vi "Lab Panel V5.24.vi"() -> ()   [LabVIEW 2013] (continued)
            n2217 = Equal?(x=w3930, y=1) -> (x = y?=w3916:bool)
            n2218 = Equal?(x=w3930, y=w3931) -> (x = y?=w3915:bool)
            n2219 = stacked-sequence {
              tunnel: w3929 -> [w3939 _ _ _ _ _ _ _ _ _]
              tunnel: w3928 -> [_ w4015 _ _ _ _ _ _ _ _]
              tunnel: w3927 -> [_ _ w4095 _ _ _ _ _ _ _]
              tunnel: w3926 -> [_ _ _ w4175 _ _ _ _ _ _]
              tunnel: w3925 -> [_ _ _ _ w4255 _ _ _ _ _]
              tunnel: w3924 -> [_ _ _ _ _ w4335 _ _ _ _]
              tunnel: w3923 -> [_ _ _ _ _ _ w4415 _ _ _]
              tunnel: w3922 -> [_ _ _ _ _ _ _ w4495 _ _]
              tunnel: w3921 -> [_ _ _ _ _ _ _ _ w4575 _]
              tunnel: w3920 -> [_ _ _ _ _ _ _ _ _ w4655]
              tunnel: w3917 -> [w3938 w4019 w4099 w4179 w4259 w4339 w4419 w4499 w4579 w4659]
              tunnel: w3916 -> [w3937 w4018 w4098 w4178 w4258 w4338 w4418 w4498 w4578 w4658]
              tunnel: w3915 -> [w3936 w4017 w4097 w4177 w4257 w4337 w4417 w4497 w4577 w4657]
              tunnel: w3914 -> [w3935 w4016 w4096 w4176 w4256 w4336 w4416 w4496 w4576 w4656]
              frame #0 {
                n2220 = case shown="True" w3939 {
                  tunnel: w3938 -> [_ w3944]
                  tunnel: w3937 -> [_ w3943]
                  tunnel: w3936 -> [_ w3941]
                  tunnel: w3935 -> [_ w3940]
                  frame False {
                  }
                  frame True {
                    n2221 = local read "DISP LAB01-1"() -> (w3945:T4)
                    n2222 = local read "SIG LAB01-1"() -> (w3946:T2)
                    n2223 = local read "ON L01-1"() -> (w3942:cluster{"amps":dbl, "volts":dbl, "pf":dbl})
                    n2224 = Unbundle(w3946) -> ("AMPS"=w3952:dbl, "VOLTS"=w3950:dbl, "PF"=w3949:dbl, "Tmp Live"=w3948:dbl, "Tmp Neut"=w3951:dbl)
                    n2225 = Unbundle(w3945) -> ("CYCLE"=w3947:dbl)  [unwired: 2 out]
                    n2226 = stacked-sequence {
                      tunnel: w3952 -> [w3956 w3975]
                      tunnel: w3951 -> [_ w3974]
                      tunnel: w3950 -> [w3955 w3973]
                      tunnel: w3949 -> [w3954 w3972]
                      tunnel: w3948 -> [_ w3971]
                      tunnel: w3947 -> [_ w3970]
                      tunnel: w3944 -> [_ w3969]
                      tunnel: w3943 -> [w3957 _]
                      tunnel: w3942 -> [w3953 w3967]
                      tunnel: w3941 -> [_ w3968]
                      tunnel: w3940 -> [_ w3963]
                      frame #0 {
                        n2227 = case shown="True" w3957 {
                          tunnel: w3956 -> [_ w3962]
                          tunnel: w3955 -> [_ w3961]
                          tunnel: w3954 -> [_ w3960]
                          tunnel: w3953 -> [_ w3958]
                          frame False {
                          }
                          frame True {
                            n2228 = Bundle(cluster=w3958, "amps"=w3962, "volts"=w3961, "pf"=w3960) -> (w3959:cluster{"amps":dbl, "volts":dbl, "pf":dbl})
                            n2229 = local write "ON L01-1"(w3959) -> ()
                          }
                        }
                      }
                      frame #1 {
                        n2230 = Unbundle(w3967) -> ("amps"=w3966:dbl, "volts"=w3965:dbl, "pf"=w3964:dbl)
                        n2231 = case shown="True" w3968 {
                          tunnel: w3975 -> [_ w3976]
                          tunnel: w3974 -> [_ w4014]
                          tunnel: w3973 -> [_ _]
                          tunnel: w3972 -> [_ _]
                          tunnel: w3971 -> [_ w4013]
                          tunnel: w3970 -> [_ w4012]
                          tunnel: w3969 -> [_ w3980]
                          tunnel: w3966 -> [_ w3977]
                          tunnel: w3965 -> [_ w4009]
                          tunnel: w3964 -> [_ w4008]
                          tunnel: w3963 -> [_ w3978]
                          frame False {
                          }
                          frame True {
                            n2232 = local read "TDMS LAB01-1"() -> (w4011:refnum<k34>)
                            n2233 = Build Array(w4009) -> (w4005:dbl[])
                            n2234 = Build Array(w4008) -> (w4004:dbl[])
                            n2235 = Build Array(w4013) -> (w4003:dbl[])
                            n2236 = Build Array(w4014) -> (w4002:dbl[])
                            n2237 = Build Array(w3977) -> (w4007:dbl[])
                            n2238 = Build Array(w3976) -> (w4006:dbl[])
                            n2239 = Build Array(w4012) -> (w4001:dbl[])
                            n2240 = Build Array("AMPS ON", "AMPS OFF", "VOLTS", "PF", "TEMP Live", "TEMP Neut", "CYCLE") -> (w3985:string[])
                            n2241 = Bundle By Name("Y"=w4007, "t0"=w3978) -> (w4000:waveform(dbl))  [unwired: 1 in]
                            n2242 = Bundle By Name("Y"=w4006, "t0"=w3978) -> (w3999:waveform(dbl))  [unwired: 1 in]
                            n2243 = Bundle By Name("Y"=w4005, "t0"=w3978) -> (w3998:waveform(dbl))  [unwired: 1 in]
                            n2244 = Bundle By Name("Y"=w4004, "t0"=w3978) -> (w3997:waveform(dbl))  [unwired: 1 in]
                            n2245 = Bundle By Name("Y"=w4003, "t0"=w3978) -> (w3996:waveform(dbl))  [unwired: 1 in]
                            n2246 = Bundle By Name("Y"=w4002, "t0"=w3978) -> (w3995:waveform(dbl))  [unwired: 1 in]
                            n2247 = Bundle By Name("Y"=w4001, "t0"=w3978) -> (w3994:waveform(dbl))  [unwired: 1 in]
                            n2248 = Build Array(w4000, w3999, w3998, w3997, w3996, w3995, w3994) -> (w3993:waveform(dbl)[])
                            n2249 = TDMS Write(0:w4011, 5:"TEST VALUES", 7:w3985, 9:w3993) -> (4:w3984:refnum<k34>, 6:w3983:string, 15:w3982:errorcluster)  [unwired: 2 in, 1 out]
                            n2250 = TDMS Write(0:w3984, 5:w3983, 7:"TIME", 9:w3980, 11:w3982) -> (15:w3979:errorcluster)  [unwired: 1 in, 3 out]
                            n2251 = local write "data file error"(w3979) -> ()
                          }
                        }
                      }
                    }
                  }
                }
              }
              frame #1 {
                n2252 = case shown="True" w4015 {
                  tunnel: w4019 -> [_ w4024]
                  tunnel: w4018 -> [_ w4023]
                  tunnel: w4017 -> [_ w4021]
                  tunnel: w4016 -> [_ w4020]
                  frame False {
                  }
                  frame True {
                    n2253 = local read "DISP LAB01-2"() -> (w4025:T4)
                    n2254 = local read "SIG LAB01-2"() -> (w4026:T2)
                    n2255 = local read "ON L01-2"() -> (w4022:cluster{"amps":dbl, "volts":dbl, "pf":dbl})
                    n2256 = Unbundle(w4026) -> ("AMPS"=w4032:dbl, "VOLTS"=w4030:dbl, "PF"=w4029:dbl, "Tmp Live"=w4028:dbl, "Tmp Neut"=w4031:dbl)
                    n2257 = Unbundle(w4025) -> ("CYCLE"=w4027:dbl)  [unwired: 2 out]
                    n2258 = stacked-sequence {
                      tunnel: w4032 -> [w4036 w4055]
                      tunnel: w4031 -> [_ w4054]
                      tunnel: w4030 -> [w4035 w4053]
                      tunnel: w4029 -> [w4034 w4052]
                      tunnel: w4028 -> [_ w4051]
                      tunnel: w4027 -> [_ w4050]
                      tunnel: w4024 -> [_ w4049]
                      tunnel: w4023 -> [w4037 _]
                      tunnel: w4022 -> [w4033 w4047]
                      tunnel: w4021 -> [_ w4048]
                      tunnel: w4020 -> [_ w4043]
                      frame #0 {
                        n2259 = case shown="True" w4037 {
                          tunnel: w4036 -> [_ w4042]
                          tunnel: w4035 -> [_ w4041]
                          tunnel: w4034 -> [_ w4040]
                          tunnel: w4033 -> [_ w4038]
                          frame False {
                          }
                          frame True {
                            n2260 = Bundle(cluster=w4038, "amps"=w4042, "volts"=w4041, "pf"=w4040) -> (w4039:cluster{"amps":dbl, "volts":dbl, "pf":dbl})
                            n2261 = local write "ON L01-2"(w4039) -> ()
                          }
                        }
                      }
                      frame #1 {
                        n2262 = Unbundle(w4047) -> ("amps"=w4046:dbl, "volts"=w4045:dbl, "pf"=w4044:dbl)
                        n2263 = case shown="True" w4048 {
                          tunnel: w4055 -> [_ w4087]
                          tunnel: w4054 -> [_ w4094]
                          tunnel: w4053 -> [_ _]
                          tunnel: w4052 -> [_ _]
                          tunnel: w4051 -> [_ w4093]
                          tunnel: w4050 -> [_ w4092]
                          tunnel: w4049 -> [_ w4057]
                          tunnel: w4046 -> [_ w4089]
                          tunnel: w4045 -> [_ w4088]
                          tunnel: w4044 -> [_ w4086]
                          tunnel: w4043 -> [_ w4078]
                          frame False {
                          }
                          frame True {
                            n2264 = local read "TDMS LAB01-2"() -> (w4091:refnum<k34>)
                            n2265 = Build Array(w4088) -> (w4083:dbl[])
                            n2266 = Build Array(w4086) -> (w4082:dbl[])
                            n2267 = Build Array(w4093) -> (w4081:dbl[])
                            n2268 = Build Array(w4094) -> (w4080:dbl[])
                            n2269 = Build Array(w4089) -> (w4085:dbl[])
                            n2270 = Build Array(w4087) -> (w4084:dbl[])
                            n2271 = Build Array(w4092) -> (w4079:dbl[])
                            n2272 = Build Array("AMPS ON", "AMPS OFF", "VOLTS", "PF", "TEMP Live", "TEMP Neut", "CYCLE") -> (w4062:string[])
                            n2273 = Bundle By Name("Y"=w4085, "t0"=w4078) -> (w4077:waveform(dbl))  [unwired: 1 in]
                            n2274 = Bundle By Name("Y"=w4084, "t0"=w4078) -> (w4076:waveform(dbl))  [unwired: 1 in]
                            n2275 = Bundle By Name("Y"=w4083, "t0"=w4078) -> (w4075:waveform(dbl))  [unwired: 1 in]
                            n2276 = Bundle By Name("Y"=w4082, "t0"=w4078) -> (w4074:waveform(dbl))  [unwired: 1 in]
                            n2277 = Bundle By Name("Y"=w4081, "t0"=w4078) -> (w4073:waveform(dbl))  [unwired: 1 in]
                            n2278 = Bundle By Name("Y"=w4080, "t0"=w4078) -> (w4072:waveform(dbl))  [unwired: 1 in]
                            n2279 = Bundle By Name("Y"=w4079, "t0"=w4078) -> (w4071:waveform(dbl))  [unwired: 1 in]
                            n2280 = Build Array(w4077, w4076, w4075, w4074, w4073, w4072, w4071) -> (w4070:waveform(dbl)[])
                            n2281 = TDMS Write(0:w4091, 5:"TEST VALUES", 7:w4062, 9:w4070) -> (4:w4061:refnum<k34>, 6:w4060:string, 15:w4059:errorcluster)  [unwired: 2 in, 1 out]
                            n2282 = TDMS Write(0:w4061, 5:w4060, 7:"TIME", 9:w4057, 11:w4059) -> (15:w4056:errorcluster)  [unwired: 1 in, 3 out]
                            n2283 = local write "data file error"(w4056) -> ()
                          }
                        }
                      }
                    }
                  }
                }
              }
              frame #2 {
                n2284 = case shown="True" w4095 {
                  tunnel: w4099 -> [_ w4104]
                  tunnel: w4098 -> [_ w4103]
                  tunnel: w4097 -> [_ w4101]
                  tunnel: w4096 -> [_ w4100]
                  frame False {
                  }
                  frame True {
                    n2285 = local read "DISP LAB02-1"() -> (w4105:T4)
                    n2286 = local read "SIG LAB02-1"() -> (w4106:T2)
                    n2287 = local read "ON L02-1"() -> (w4102:cluster{"amps":dbl, "volts":dbl, "pf":dbl})
                    n2288 = Unbundle(w4106) -> ("AMPS"=w4112:dbl, "VOLTS"=w4110:dbl, "PF"=w4109:dbl, "Tmp Live"=w4108:dbl, "Tmp Neut"=w4111:dbl)
                    n2289 = Unbundle(w4105) -> ("CYCLE"=w4107:dbl)  [unwired: 2 out]
                    n2290 = stacked-sequence {
                      tunnel: w4112 -> [w4116 w4135]
                      tunnel: w4111 -> [_ w4134]
                      tunnel: w4110 -> [w4115 w4133]
                      tunnel: w4109 -> [w4114 w4132]
                      tunnel: w4108 -> [_ w4131]
                      tunnel: w4107 -> [_ w4130]
                      tunnel: w4104 -> [_ w4129]
                      tunnel: w4103 -> [w4117 _]
                      tunnel: w4102 -> [w4113 w4127]
                      tunnel: w4101 -> [_ w4128]
                      tunnel: w4100 -> [_ w4123]
                      frame #0 {
                        n2291 = case shown="True" w4117 {
                          tunnel: w4116 -> [_ w4122]
                          tunnel: w4115 -> [_ w4121]
                          tunnel: w4114 -> [_ w4120]
                          tunnel: w4113 -> [_ w4118]
                          frame False {
                          }
                          frame True {
                            n2292 = Bundle(cluster=w4118, "amps"=w4122, "volts"=w4121, "pf"=w4120) -> (w4119:cluster{"amps":dbl, "volts":dbl, "pf":dbl})
                            n2293 = local write "ON L02-1"(w4119) -> ()
                          }
                        }
                      }
                      frame #1 {
                        n2294 = Unbundle(w4127) -> ("amps"=w4126:dbl, "volts"=w4125:dbl, "pf"=w4124:dbl)
                        n2295 = case shown="True" w4128 {
                          tunnel: w4135 -> [_ w4167]
                          tunnel: w4134 -> [_ w4174]
                          tunnel: w4133 -> [_ _]
                          tunnel: w4132 -> [_ _]
                          tunnel: w4131 -> [_ w4173]
                          tunnel: w4130 -> [_ w4172]
                          tunnel: w4129 -> [_ w4137]
                          tunnel: w4126 -> [_ w4169]
                          tunnel: w4125 -> [_ w4168]
                          tunnel: w4124 -> [_ w4166]
                          tunnel: w4123 -> [_ w4158]
                          frame False {
                          }
                          frame True {
                            n2296 = local read "TDMS LAB02-1"() -> (w4171:refnum<k34>)
                            n2297 = Build Array(w4168) -> (w4163:dbl[])
                            n2298 = Build Array(w4166) -> (w4162:dbl[])
                            n2299 = Build Array(w4173) -> (w4161:dbl[])
                            n2300 = Build Array(w4174) -> (w4160:dbl[])
                            n2301 = Build Array(w4169) -> (w4165:dbl[])
                            n2302 = Build Array(w4167) -> (w4164:dbl[])
                            n2303 = Build Array(w4172) -> (w4159:dbl[])
                            n2304 = Build Array("AMPS ON", "AMPS OFF", "VOLTS", "PF", "TEMP Live", "TEMP Neut", "CYCLE") -> (w4142:string[])
                            n2305 = Bundle By Name("Y"=w4165, "t0"=w4158) -> (w4157:waveform(dbl))  [unwired: 1 in]
                            n2306 = Bundle By Name("Y"=w4164, "t0"=w4158) -> (w4156:waveform(dbl))  [unwired: 1 in]
                            n2307 = Bundle By Name("Y"=w4163, "t0"=w4158) -> (w4155:waveform(dbl))  [unwired: 1 in]
                            n2308 = Bundle By Name("Y"=w4162, "t0"=w4158) -> (w4154:waveform(dbl))  [unwired: 1 in]
                            n2309 = Bundle By Name("Y"=w4161, "t0"=w4158) -> (w4153:waveform(dbl))  [unwired: 1 in]
                            n2310 = Bundle By Name("Y"=w4160, "t0"=w4158) -> (w4152:waveform(dbl))  [unwired: 1 in]
                            n2311 = Bundle By Name("Y"=w4159, "t0"=w4158) -> (w4151:waveform(dbl))  [unwired: 1 in]
                            n2312 = Build Array(w4157, w4156, w4155, w4154, w4153, w4152, w4151) -> (w4150:waveform(dbl)[])
                            n2313 = TDMS Write(0:w4171, 5:"TEST VALUES", 7:w4142, 9:w4150) -> (4:w4141:refnum<k34>, 6:w4140:string, 15:w4139:errorcluster)  [unwired: 2 in, 1 out]
                            n2314 = TDMS Write(0:w4141, 5:w4140, 7:"TIME", 9:w4137, 11:w4139) -> (15:w4136:errorcluster)  [unwired: 1 in, 3 out]
                            n2315 = local write "data file error"(w4136) -> ()
                          }
                        }
                      }
                    }
                  }
                }
              }
              frame #3 {
                n2316 = case shown="True" w4175 {
                  tunnel: w4179 -> [_ w4184]
                  tunnel: w4178 -> [_ w4183]
                  tunnel: w4177 -> [_ w4181]
                  tunnel: w4176 -> [_ w4180]
                  frame False {
                  }
                  frame True {
                    n2317 = local read "DISP LAB02-2"() -> (w4185:T4)
                    n2318 = local read "SIG LAB02-2"() -> (w4186:T2)
                    n2319 = local read "ON L02-2"() -> (w4182:cluster{"amps":dbl, "volts":dbl, "pf":dbl})
                    n2320 = Unbundle(w4186) -> ("AMPS"=w4192:dbl, "VOLTS"=w4190:dbl, "PF"=w4189:dbl, "Tmp Live"=w4188:dbl, "Tmp Neut"=w4191:dbl)
                    n2321 = Unbundle(w4185) -> ("CYCLE"=w4187:dbl)  [unwired: 2 out]
                    n2322 = stacked-sequence {
                      tunnel: w4192 -> [w4196 w4215]
                      tunnel: w4191 -> [_ w4214]
                      tunnel: w4190 -> [w4195 w4213]
                      tunnel: w4189 -> [w4194 w4212]
                      tunnel: w4188 -> [_ w4211]
                      tunnel: w4187 -> [_ w4210]
                      tunnel: w4184 -> [_ w4209]
                      tunnel: w4183 -> [w4197 _]
                      tunnel: w4182 -> [w4193 w4207]
                      tunnel: w4181 -> [_ w4208]
                      tunnel: w4180 -> [_ w4203]
                      frame #0 {
                        n2323 = case shown="True" w4197 {
                          tunnel: w4196 -> [_ w4202]
                          tunnel: w4195 -> [_ w4201]
                          tunnel: w4194 -> [_ w4200]
                          tunnel: w4193 -> [_ w4198]
                          frame False {
                          }
                          frame True {
                            n2324 = Bundle(cluster=w4198, "amps"=w4202, "volts"=w4201, "pf"=w4200) -> (w4199:cluster{"amps":dbl, "volts":dbl, "pf":dbl})
                            n2325 = local write "ON L02-2"(w4199) -> ()
                          }
                        }
                      }
                      frame #1 {
                        n2326 = Unbundle(w4207) -> ("amps"=w4206:dbl, "volts"=w4205:dbl, "pf"=w4204:dbl)
                        n2327 = case shown="True" w4208 {
                          tunnel: w4215 -> [_ w4247]
                          tunnel: w4214 -> [_ w4254]
                          tunnel: w4213 -> [_ _]
                          tunnel: w4212 -> [_ _]
                          tunnel: w4211 -> [_ w4253]
                          tunnel: w4210 -> [_ w4252]
                          tunnel: w4209 -> [_ w4217]
                          tunnel: w4206 -> [_ w4249]
                          tunnel: w4205 -> [_ w4248]
                          tunnel: w4204 -> [_ w4246]
                          tunnel: w4203 -> [_ w4238]
                          frame False {
                          }
                          frame True {
                            n2328 = local read "TDMS LAB02-2"() -> (w4251:refnum<k34>)
                            n2329 = Build Array(w4248) -> (w4243:dbl[])
                            n2330 = Build Array(w4246) -> (w4242:dbl[])
                            n2331 = Build Array(w4253) -> (w4241:dbl[])
                            n2332 = Build Array(w4254) -> (w4240:dbl[])
                            n2333 = Build Array(w4249) -> (w4245:dbl[])
                            n2334 = Build Array(w4247) -> (w4244:dbl[])
                            n2335 = Build Array(w4252) -> (w4239:dbl[])
                            n2336 = Build Array("AMPS ON", "AMPS OFF", "VOLTS", "PF", "TEMP Live", "TEMP Neut", "CYCLE") -> (w4222:string[])
                            n2337 = Bundle By Name("Y"=w4245, "t0"=w4238) -> (w4237:waveform(dbl))  [unwired: 1 in]
                            n2338 = Bundle By Name("Y"=w4244, "t0"=w4238) -> (w4236:waveform(dbl))  [unwired: 1 in]
                            n2339 = Bundle By Name("Y"=w4243, "t0"=w4238) -> (w4235:waveform(dbl))  [unwired: 1 in]
                            n2340 = Bundle By Name("Y"=w4242, "t0"=w4238) -> (w4234:waveform(dbl))  [unwired: 1 in]
                            n2341 = Bundle By Name("Y"=w4241, "t0"=w4238) -> (w4233:waveform(dbl))  [unwired: 1 in]
                            n2342 = Bundle By Name("Y"=w4240, "t0"=w4238) -> (w4232:waveform(dbl))  [unwired: 1 in]
                            n2343 = Bundle By Name("Y"=w4239, "t0"=w4238) -> (w4231:waveform(dbl))  [unwired: 1 in]
                            n2344 = Build Array(w4237, w4236, w4235, w4234, w4233, w4232, w4231) -> (w4230:waveform(dbl)[])
                            n2345 = TDMS Write(0:w4251, 5:"TEST VALUES", 7:w4222, 9:w4230) -> (4:w4221:refnum<k34>, 6:w4220:string, 15:w4219:errorcluster)  [unwired: 2 in, 1 out]
                            n2346 = TDMS Write(0:w4221, 5:w4220, 7:"TIME", 9:w4217, 11:w4219) -> (15:w4216:errorcluster)  [unwired: 1 in, 3 out]
                            n2347 = local write "data file error"(w4216) -> ()
                          }
                        }
                      }
                    }
                  }
                }
              }
              frame #4 {
                n2348 = case shown="True" w4255 {
                  tunnel: w4259 -> [_ w4264]
                  tunnel: w4258 -> [_ w4263]
                  tunnel: w4257 -> [_ w4261]
                  tunnel: w4256 -> [_ w4260]
                  frame False {
                  }
                  frame True {
                    n2349 = local read "DISP LAB03-1"() -> (w4265:T4)
                    n2350 = local read "SIG LAB03-1"() -> (w4266:T2)
                    n2351 = local read "ON L03-1"() -> (w4262:cluster{"amps":dbl, "volts":dbl, "pf":dbl})
                    n2352 = Unbundle(w4266) -> ("AMPS"=w4272:dbl, "VOLTS"=w4270:dbl, "PF"=w4269:dbl, "Tmp Live"=w4268:dbl, "Tmp Neut"=w4271:dbl)
                    n2353 = Unbundle(w4265) -> ("CYCLE"=w4267:dbl)  [unwired: 2 out]
                    n2354 = stacked-sequence {
                      tunnel: w4272 -> [w4276 w4295]
                      tunnel: w4271 -> [_ w4294]
                      tunnel: w4270 -> [w4275 w4293]
                      tunnel: w4269 -> [w4274 w4292]
                      tunnel: w4268 -> [_ w4291]
                      tunnel: w4267 -> [_ w4290]
                      tunnel: w4264 -> [_ w4289]
                      tunnel: w4263 -> [w4277 _]
                      tunnel: w4262 -> [w4273 w4287]
                      tunnel: w4261 -> [_ w4288]
                      tunnel: w4260 -> [_ w4283]
                      frame #0 {
                        n2355 = case shown="True" w4277 {
                          tunnel: w4276 -> [_ w4282]
                          tunnel: w4275 -> [_ w4281]
                          tunnel: w4274 -> [_ w4280]
                          tunnel: w4273 -> [_ w4278]
                          frame False {
                          }
                          frame True {
                            n2356 = Bundle(cluster=w4278, "amps"=w4282, "volts"=w4281, "pf"=w4280) -> (w4279:cluster{"amps":dbl, "volts":dbl, "pf":dbl})
                            n2357 = local write "ON L03-1"(w4279) -> ()
                          }
                        }
                      }
                      frame #1 {
                        n2358 = Unbundle(w4287) -> ("amps"=w4286:dbl, "volts"=w4285:dbl, "pf"=w4284:dbl)
                        n2359 = case shown="True" w4288 {
                          tunnel: w4295 -> [_ w4327]
                          tunnel: w4294 -> [_ w4334]
                          tunnel: w4293 -> [_ _]
                          tunnel: w4292 -> [_ _]
                          tunnel: w4291 -> [_ w4333]
                          tunnel: w4290 -> [_ w4332]
                          tunnel: w4289 -> [_ w4297]
                          tunnel: w4286 -> [_ w4329]
                          tunnel: w4285 -> [_ w4328]
                          tunnel: w4284 -> [_ w4326]
                          tunnel: w4283 -> [_ w4318]
                          frame False {
                          }
                          frame True {
                            n2360 = local read "TDMS LAB03-1"() -> (w4331:refnum<k34>)
                            n2361 = Build Array(w4328) -> (w4323:dbl[])
                            n2362 = Build Array(w4326) -> (w4322:dbl[])
                            n2363 = Build Array(w4333) -> (w4321:dbl[])
                            n2364 = Build Array(w4334) -> (w4320:dbl[])
                            n2365 = Build Array(w4329) -> (w4325:dbl[])
                            n2366 = Build Array(w4327) -> (w4324:dbl[])
                            n2367 = Build Array(w4332) -> (w4319:dbl[])
                            n2368 = Build Array("AMPS ON", "AMPS OFF", "VOLTS", "PF", "TEMP Live", "TEMP Neut", "CYCLE") -> (w4302:string[])
                            n2369 = Bundle By Name("Y"=w4325, "t0"=w4318) -> (w4317:waveform(dbl))  [unwired: 1 in]
                            n2370 = Bundle By Name("Y"=w4324, "t0"=w4318) -> (w4316:waveform(dbl))  [unwired: 1 in]
                            n2371 = Bundle By Name("Y"=w4323, "t0"=w4318) -> (w4315:waveform(dbl))  [unwired: 1 in]
                            n2372 = Bundle By Name("Y"=w4322, "t0"=w4318) -> (w4314:waveform(dbl))  [unwired: 1 in]
                            n2373 = Bundle By Name("Y"=w4321, "t0"=w4318) -> (w4313:waveform(dbl))  [unwired: 1 in]
                            n2374 = Bundle By Name("Y"=w4320, "t0"=w4318) -> (w4312:waveform(dbl))  [unwired: 1 in]
                            n2375 = Bundle By Name("Y"=w4319, "t0"=w4318) -> (w4311:waveform(dbl))  [unwired: 1 in]
                            n2376 = Build Array(w4317, w4316, w4315, w4314, w4313, w4312, w4311) -> (w4310:waveform(dbl)[])
                            n2377 = TDMS Write(0:w4331, 5:"TEST VALUES", 7:w4302, 9:w4310) -> (4:w4301:refnum<k34>, 6:w4300:string, 15:w4299:errorcluster)  [unwired: 2 in, 1 out]
                            n2378 = TDMS Write(0:w4301, 5:w4300, 7:"TIME", 9:w4297, 11:w4299) -> (15:w4296:errorcluster)  [unwired: 1 in, 3 out]
                            n2379 = local write "data file error"(w4296) -> ()
                          }
                        }
                      }
                    }
                  }
                }
              }
              frame #5 {
                n2380 = case shown="True" w4335 {
                  tunnel: w4339 -> [_ w4344]
                  tunnel: w4338 -> [_ w4343]
                  tunnel: w4337 -> [_ w4341]
                  tunnel: w4336 -> [_ w4340]
                  frame False {
                  }
                  frame True {
                    n2381 = local read "DISP LAB03-2"() -> (w4345:T4)
                    n2382 = local read "SIG LAB03-2"() -> (w4346:T2)
                    n2383 = local read "ON L03-2"() -> (w4342:cluster{"amps":dbl, "volts":dbl, "pf":dbl})
                    n2384 = Unbundle(w4346) -> ("AMPS"=w4352:dbl, "VOLTS"=w4350:dbl, "PF"=w4349:dbl, "Tmp Live"=w4348:dbl, "Tmp Neut"=w4351:dbl)
                    n2385 = Unbundle(w4345) -> ("CYCLE"=w4347:dbl)  [unwired: 2 out]
                    n2386 = stacked-sequence {
                      tunnel: w4352 -> [w4356 w4375]
                      tunnel: w4351 -> [_ w4374]
                      tunnel: w4350 -> [w4355 w4373]
                      tunnel: w4349 -> [w4354 w4372]
                      tunnel: w4348 -> [_ w4371]
                      tunnel: w4347 -> [_ w4370]
                      tunnel: w4344 -> [_ w4369]
                      tunnel: w4343 -> [w4357 _]
                      tunnel: w4342 -> [w4353 w4367]
                      tunnel: w4341 -> [_ w4368]
                      tunnel: w4340 -> [_ w4363]
                      frame #0 {
                        n2387 = case shown="True" w4357 {
                          tunnel: w4356 -> [_ w4362]
                          tunnel: w4355 -> [_ w4361]
                          tunnel: w4354 -> [_ w4360]
                          tunnel: w4353 -> [_ w4358]
                          frame False {
                          }
                          frame True {
                            n2388 = Bundle(cluster=w4358, "amps"=w4362, "volts"=w4361, "pf"=w4360) -> (w4359:cluster{"amps":dbl, "volts":dbl, "pf":dbl})
                            n2389 = local write "ON L03-2"(w4359) -> ()
                          }
                        }
                      }
                      frame #1 {
                        n2390 = Unbundle(w4367) -> ("amps"=w4366:dbl, "volts"=w4365:dbl, "pf"=w4364:dbl)
                        n2391 = case shown="True" w4368 {
                          tunnel: w4375 -> [_ w4407]
                          tunnel: w4374 -> [_ w4414]
                          tunnel: w4373 -> [_ _]
                          tunnel: w4372 -> [_ _]
                          tunnel: w4371 -> [_ w4413]
                          tunnel: w4370 -> [_ w4412]
                          tunnel: w4369 -> [_ w4377]
                          tunnel: w4366 -> [_ w4409]
                          tunnel: w4365 -> [_ w4408]
                          tunnel: w4364 -> [_ w4406]
                          tunnel: w4363 -> [_ w4398]
                          frame False {
                          }
                          frame True {
                            n2392 = local read "TDMS LAB03-2"() -> (w4411:refnum<k34>)
                            n2393 = Build Array(w4408) -> (w4403:dbl[])
                            n2394 = Build Array(w4406) -> (w4402:dbl[])
                            n2395 = Build Array(w4413) -> (w4401:dbl[])
                            n2396 = Build Array(w4414) -> (w4400:dbl[])
                            n2397 = Build Array(w4409) -> (w4405:dbl[])
                            n2398 = Build Array(w4407) -> (w4404:dbl[])
                            n2399 = Build Array(w4412) -> (w4399:dbl[])
                            n2400 = Build Array("AMPS ON", "AMPS OFF", "VOLTS", "PF", "TEMP Live", "TEMP Neut", "CYCLE") -> (w4382:string[])
                            n2401 = Bundle By Name("Y"=w4405, "t0"=w4398) -> (w4397:waveform(dbl))  [unwired: 1 in]
                            n2402 = Bundle By Name("Y"=w4404, "t0"=w4398) -> (w4396:waveform(dbl))  [unwired: 1 in]
                            n2403 = Bundle By Name("Y"=w4403, "t0"=w4398) -> (w4395:waveform(dbl))  [unwired: 1 in]
                            n2404 = Bundle By Name("Y"=w4402, "t0"=w4398) -> (w4394:waveform(dbl))  [unwired: 1 in]
                            n2405 = Bundle By Name("Y"=w4401, "t0"=w4398) -> (w4393:waveform(dbl))  [unwired: 1 in]
                            n2406 = Bundle By Name("Y"=w4400, "t0"=w4398) -> (w4392:waveform(dbl))  [unwired: 1 in]
                            n2407 = Bundle By Name("Y"=w4399, "t0"=w4398) -> (w4391:waveform(dbl))  [unwired: 1 in]
                            n2408 = Build Array(w4397, w4396, w4395, w4394, w4393, w4392, w4391) -> (w4390:waveform(dbl)[])
                            n2409 = TDMS Write(0:w4411, 5:"TEST VALUES", 7:w4382, 9:w4390) -> (4:w4381:refnum<k34>, 6:w4380:string, 15:w4379:errorcluster)  [unwired: 2 in, 1 out]
                            n2410 = TDMS Write(0:w4381, 5:w4380, 7:"TIME", 9:w4377, 11:w4379) -> (15:w4376:errorcluster)  [unwired: 1 in, 3 out]
                            n2411 = local write "data file error"(w4376) -> ()
                          }
                        }
                      }
                    }
                  }
                }
              }
              frame #6 {
                n2412 = case shown="True" w4415 {
                  tunnel: w4419 -> [_ w4424]
                  tunnel: w4418 -> [_ w4423]
                  tunnel: w4417 -> [_ w4421]
                  tunnel: w4416 -> [_ w4420]
                  frame False {
                  }
                  frame True {
                    n2413 = local read "DISP LAB04-1"() -> (w4425:T4)
                    n2414 = local read "SIG LAB04-1"() -> (w4426:T2)
                    n2415 = local read "ON L04-1"() -> (w4422:cluster{"amps":dbl, "volts":dbl, "pf":dbl})
                    n2416 = Unbundle(w4426) -> ("AMPS"=w4432:dbl, "VOLTS"=w4430:dbl, "PF"=w4429:dbl, "Tmp Live"=w4428:dbl, "Tmp Neut"=w4431:dbl)
                    n2417 = Unbundle(w4425) -> ("CYCLE"=w4427:dbl)  [unwired: 2 out]
                    n2418 = stacked-sequence {
                      tunnel: w4432 -> [w4436 w4455]
                      tunnel: w4431 -> [_ w4454]
                      tunnel: w4430 -> [w4435 w4453]
                      tunnel: w4429 -> [w4434 w4452]
                      tunnel: w4428 -> [_ w4451]
                      tunnel: w4427 -> [_ w4450]
                      tunnel: w4424 -> [_ w4449]
                      tunnel: w4423 -> [w4437 _]
                      tunnel: w4422 -> [w4433 w4447]
                      tunnel: w4421 -> [_ w4448]
                      tunnel: w4420 -> [_ w4443]
                      frame #0 {
                        n2419 = case shown="True" w4437 {
                          tunnel: w4436 -> [_ w4442]
                          tunnel: w4435 -> [_ w4441]
                          tunnel: w4434 -> [_ w4440]
                          tunnel: w4433 -> [_ w4438]
                          frame False {
                          }
                          frame True {
                            n2420 = Bundle(cluster=w4438, "amps"=w4442, "volts"=w4441, "pf"=w4440) -> (w4439:cluster{"amps":dbl, "volts":dbl, "pf":dbl})
                            n2421 = local write "ON L04-1"(w4439) -> ()
                          }
                        }
                      }
                      frame #1 {
                        n2422 = Unbundle(w4447) -> ("amps"=w4446:dbl, "volts"=w4445:dbl, "pf"=w4444:dbl)
                        n2423 = case shown="True" w4448 {
                          tunnel: w4455 -> [_ w4487]
                          tunnel: w4454 -> [_ w4494]
                          tunnel: w4453 -> [_ _]
                          tunnel: w4452 -> [_ _]
                          tunnel: w4451 -> [_ w4493]
                          tunnel: w4450 -> [_ w4492]
                          tunnel: w4449 -> [_ w4457]
                          tunnel: w4446 -> [_ w4489]
                          tunnel: w4445 -> [_ w4488]
                          tunnel: w4444 -> [_ w4486]
                          tunnel: w4443 -> [_ w4478]
                          frame False {
                          }
                          frame True {
                            n2424 = local read "TDMS LAB04-1"() -> (w4491:refnum<k34>)
                            n2425 = Build Array(w4488) -> (w4483:dbl[])
                            n2426 = Build Array(w4486) -> (w4482:dbl[])
                            n2427 = Build Array(w4493) -> (w4481:dbl[])
                            n2428 = Build Array(w4494) -> (w4480:dbl[])
                            n2429 = Build Array(w4489) -> (w4485:dbl[])
                            n2430 = Build Array(w4487) -> (w4484:dbl[])
                            n2431 = Build Array(w4492) -> (w4479:dbl[])
                            n2432 = Build Array("AMPS ON", "AMPS OFF", "VOLTS", "PF", "TEMP Live", "TEMP Neut", "CYCLE") -> (w4462:string[])
                            n2433 = Bundle By Name("Y"=w4485, "t0"=w4478) -> (w4477:waveform(dbl))  [unwired: 1 in]
                            n2434 = Bundle By Name("Y"=w4484, "t0"=w4478) -> (w4476:waveform(dbl))  [unwired: 1 in]
                            n2435 = Bundle By Name("Y"=w4483, "t0"=w4478) -> (w4475:waveform(dbl))  [unwired: 1 in]
                            n2436 = Bundle By Name("Y"=w4482, "t0"=w4478) -> (w4474:waveform(dbl))  [unwired: 1 in]
                            n2437 = Bundle By Name("Y"=w4481, "t0"=w4478) -> (w4473:waveform(dbl))  [unwired: 1 in]
                            n2438 = Bundle By Name("Y"=w4480, "t0"=w4478) -> (w4472:waveform(dbl))  [unwired: 1 in]
                            n2439 = Bundle By Name("Y"=w4479, "t0"=w4478) -> (w4471:waveform(dbl))  [unwired: 1 in]
                            n2440 = Build Array(w4477, w4476, w4475, w4474, w4473, w4472, w4471) -> (w4470:waveform(dbl)[])
                            n2441 = TDMS Write(0:w4491, 5:"TEST VALUES", 7:w4462, 9:w4470) -> (4:w4461:refnum<k34>, 6:w4460:string, 15:w4459:errorcluster)  [unwired: 2 in, 1 out]
                            n2442 = TDMS Write(0:w4461, 5:w4460, 7:"TIME", 9:w4457, 11:w4459) -> (15:w4456:errorcluster)  [unwired: 1 in, 3 out]
                            n2443 = local write "data file error"(w4456) -> ()
                          }
                        }
                      }
                    }
                  }
                }
              }
              frame #7 {
                n2444 = case shown="True" w4495 {
                  tunnel: w4499 -> [_ w4504]
                  tunnel: w4498 -> [_ w4503]
                  tunnel: w4497 -> [_ w4501]
                  tunnel: w4496 -> [_ w4500]
                  frame False {
                  }
                  frame True {
                    n2445 = local read "DISP LAB04-2"() -> (w4505:T4)
                    n2446 = local read "SIG LAB04-2"() -> (w4506:T2)
                    n2447 = local read "ON L04-2"() -> (w4502:cluster{"amps":dbl, "volts":dbl, "pf":dbl})
                    n2448 = Unbundle(w4506) -> ("AMPS"=w4512:dbl, "VOLTS"=w4510:dbl, "PF"=w4509:dbl, "Tmp Live"=w4508:dbl, "Tmp Neut"=w4511:dbl)
                    n2449 = Unbundle(w4505) -> ("CYCLE"=w4507:dbl)  [unwired: 2 out]
                    n2450 = stacked-sequence {
                      tunnel: w4512 -> [w4516 w4535]
                      tunnel: w4511 -> [_ w4534]
                      tunnel: w4510 -> [w4515 w4533]
                      tunnel: w4509 -> [w4514 w4532]
                      tunnel: w4508 -> [_ w4531]
                      tunnel: w4507 -> [_ w4530]
                      tunnel: w4504 -> [_ w4529]
                      tunnel: w4503 -> [w4517 _]
                      tunnel: w4502 -> [w4513 w4527]
                      tunnel: w4501 -> [_ w4528]
                      tunnel: w4500 -> [_ w4523]
                      frame #0 {
                        n2451 = case shown="True" w4517 {
                          tunnel: w4516 -> [_ w4522]
                          tunnel: w4515 -> [_ w4521]
                          tunnel: w4514 -> [_ w4520]
                          tunnel: w4513 -> [_ w4518]
                          frame False {
                          }
                          frame True {
                            n2452 = Bundle(cluster=w4518, "amps"=w4522, "volts"=w4521, "pf"=w4520) -> (w4519:cluster{"amps":dbl, "volts":dbl, "pf":dbl})
                            n2453 = local write "ON L04-2"(w4519) -> ()
                          }
                        }
                      }
                      frame #1 {
                        n2454 = Unbundle(w4527) -> ("amps"=w4526:dbl, "volts"=w4525:dbl, "pf"=w4524:dbl)
                        n2455 = case shown="True" w4528 {
                          tunnel: w4535 -> [_ w4567]
                          tunnel: w4534 -> [_ w4574]
                          tunnel: w4533 -> [_ _]
                          tunnel: w4532 -> [_ _]
                          tunnel: w4531 -> [_ w4573]
                          tunnel: w4530 -> [_ w4572]
                          tunnel: w4529 -> [_ w4537]
                          tunnel: w4526 -> [_ w4569]
                          tunnel: w4525 -> [_ w4568]
                          tunnel: w4524 -> [_ w4566]
                          tunnel: w4523 -> [_ w4558]
                          frame False {
                          }
                          frame True {
                            n2456 = local read "TDMS LAB04-2"() -> (w4571:refnum<k34>)
                            n2457 = Build Array(w4568) -> (w4563:dbl[])
                            n2458 = Build Array(w4566) -> (w4562:dbl[])
                            n2459 = Build Array(w4573) -> (w4561:dbl[])
                            n2460 = Build Array(w4574) -> (w4560:dbl[])
                            n2461 = Build Array(w4569) -> (w4565:dbl[])
                            n2462 = Build Array(w4567) -> (w4564:dbl[])
                            n2463 = Build Array(w4572) -> (w4559:dbl[])
                            n2464 = Build Array("AMPS ON", "AMPS OFF", "VOLTS", "PF", "TEMP Live", "TEMP Neut", "CYCLE") -> (w4542:string[])
                            n2465 = Bundle By Name("Y"=w4565, "t0"=w4558) -> (w4557:waveform(dbl))  [unwired: 1 in]
                            n2466 = Bundle By Name("Y"=w4564, "t0"=w4558) -> (w4556:waveform(dbl))  [unwired: 1 in]
                            n2467 = Bundle By Name("Y"=w4563, "t0"=w4558) -> (w4555:waveform(dbl))  [unwired: 1 in]
                            n2468 = Bundle By Name("Y"=w4562, "t0"=w4558) -> (w4554:waveform(dbl))  [unwired: 1 in]
                            n2469 = Bundle By Name("Y"=w4561, "t0"=w4558) -> (w4553:waveform(dbl))  [unwired: 1 in]
                            n2470 = Bundle By Name("Y"=w4560, "t0"=w4558) -> (w4552:waveform(dbl))  [unwired: 1 in]
                            n2471 = Bundle By Name("Y"=w4559, "t0"=w4558) -> (w4551:waveform(dbl))  [unwired: 1 in]
                            n2472 = Build Array(w4557, w4556, w4555, w4554, w4553, w4552, w4551) -> (w4550:waveform(dbl)[])
                            n2473 = TDMS Write(0:w4571, 5:"TEST VALUES", 7:w4542, 9:w4550) -> (4:w4541:refnum<k34>, 6:w4540:string, 15:w4539:errorcluster)  [unwired: 2 in, 1 out]
                            n2474 = TDMS Write(0:w4541, 5:w4540, 7:"TIME", 9:w4537, 11:w4539) -> (15:w4536:errorcluster)  [unwired: 1 in, 3 out]
                            n2475 = local write "data file error"(w4536) -> ()
                          }
                        }
                      }
                    }
                  }
                }
              }
              frame #8 {
                n2476 = case shown="True" w4575 {
                  tunnel: w4579 -> [_ w4584]
                  tunnel: w4578 -> [_ w4583]
                  tunnel: w4577 -> [_ w4581]
                  tunnel: w4576 -> [_ w4580]
                  frame False {
                  }
                  frame True {
                    n2477 = local read "DISP LAB05-1"() -> (w4585:T4)
                    n2478 = local read "SIG LAB05-1"() -> (w4586:T2)
                    n2479 = local read "ON L05-1"() -> (w4582:cluster{"amps":dbl, "volts":dbl, "pf":dbl})
                    n2480 = Unbundle(w4586) -> ("AMPS"=w4592:dbl, "VOLTS"=w4590:dbl, "PF"=w4589:dbl, "Tmp Live"=w4588:dbl, "Tmp Neut"=w4591:dbl)
                    n2481 = Unbundle(w4585) -> ("CYCLE"=w4587:dbl)  [unwired: 2 out]
                    n2482 = stacked-sequence {
                      tunnel: w4592 -> [w4596 w4615]
                      tunnel: w4591 -> [_ w4614]
                      tunnel: w4590 -> [w4595 w4613]
                      tunnel: w4589 -> [w4594 w4612]
                      tunnel: w4588 -> [_ w4611]
                      tunnel: w4587 -> [_ w4610]
                      tunnel: w4584 -> [_ w4609]
                      tunnel: w4583 -> [w4597 _]
                      tunnel: w4582 -> [w4593 w4607]
                      tunnel: w4581 -> [_ w4608]
                      tunnel: w4580 -> [_ w4603]
                      frame #0 {
                        n2483 = case shown="True" w4597 {
                          tunnel: w4596 -> [_ w4602]
                          tunnel: w4595 -> [_ w4601]
                          tunnel: w4594 -> [_ w4600]
                          tunnel: w4593 -> [_ w4598]
                          frame False {
                          }
                          frame True {
                            n2484 = Bundle(cluster=w4598, "amps"=w4602, "volts"=w4601, "pf"=w4600) -> (w4599:cluster{"amps":dbl, "volts":dbl, "pf":dbl})
                            n2485 = local write "ON L05-1"(w4599) -> ()
                          }
                        }
                      }
                      frame #1 {
                        n2486 = Unbundle(w4607) -> ("amps"=w4606:dbl, "volts"=w4605:dbl, "pf"=w4604:dbl)
                        n2487 = case shown="True" w4608 {
                          tunnel: w4615 -> [_ w4647]
                          tunnel: w4614 -> [_ w4654]
                          tunnel: w4613 -> [_ _]
                          tunnel: w4612 -> [_ _]
                          tunnel: w4611 -> [_ w4653]
                          tunnel: w4610 -> [_ w4652]
                          tunnel: w4609 -> [_ w4617]
                          tunnel: w4606 -> [_ w4649]
                          tunnel: w4605 -> [_ w4648]
                          tunnel: w4604 -> [_ w4646]
                          tunnel: w4603 -> [_ w4638]
                          frame False {
                          }
                          frame True {
                            n2488 = local read "TDMS LAB05-1"() -> (w4651:refnum<k34>)
                            n2489 = Build Array(w4648) -> (w4643:dbl[])
                            n2490 = Build Array(w4646) -> (w4642:dbl[])
                            n2491 = Build Array(w4653) -> (w4641:dbl[])
                            n2492 = Build Array(w4654) -> (w4640:dbl[])
                            n2493 = Build Array(w4649) -> (w4645:dbl[])
                            n2494 = Build Array(w4647) -> (w4644:dbl[])
                            n2495 = Build Array(w4652) -> (w4639:dbl[])
                            n2496 = Build Array("AMPS ON", "AMPS OFF", "VOLTS", "PF", "TEMP Live", "TEMP Neut", "CYCLE") -> (w4622:string[])
                            n2497 = Bundle By Name("Y"=w4645, "t0"=w4638) -> (w4637:waveform(dbl))  [unwired: 1 in]
                            n2498 = Bundle By Name("Y"=w4644, "t0"=w4638) -> (w4636:waveform(dbl))  [unwired: 1 in]
                            n2499 = Bundle By Name("Y"=w4643, "t0"=w4638) -> (w4635:waveform(dbl))  [unwired: 1 in]
                            n2500 = Bundle By Name("Y"=w4642, "t0"=w4638) -> (w4634:waveform(dbl))  [unwired: 1 in]
                            n2501 = Bundle By Name("Y"=w4641, "t0"=w4638) -> (w4633:waveform(dbl))  [unwired: 1 in]
                            n2502 = Bundle By Name("Y"=w4640, "t0"=w4638) -> (w4632:waveform(dbl))  [unwired: 1 in]
                            n2503 = Bundle By Name("Y"=w4639, "t0"=w4638) -> (w4631:waveform(dbl))  [unwired: 1 in]
                            n2504 = Build Array(w4637, w4636, w4635, w4634, w4633, w4632, w4631) -> (w4630:waveform(dbl)[])
                            n2505 = TDMS Write(0:w4651, 5:"TEST VALUES", 7:w4622, 9:w4630) -> (4:w4621:refnum<k34>, 6:w4620:string, 15:w4619:errorcluster)  [unwired: 2 in, 1 out]
                            n2506 = TDMS Write(0:w4621, 5:w4620, 7:"TIME", 9:w4617, 11:w4619) -> (15:w4616:errorcluster)  [unwired: 1 in, 3 out]
                            n2507 = local write "data file error"(w4616) -> ()
                          }
                        }
                      }
                    }
                  }
                }
              }
              frame #9 {
                n2508 = case shown="True" w4655 {
                  tunnel: w4659 -> [_ w4664]
                  tunnel: w4658 -> [_ w4663]
                  tunnel: w4657 -> [_ w4661]
                  tunnel: w4656 -> [_ w4660]
                  frame False {
                  }
                  frame True {
                    n2509 = local read "DISP LAB05-2"() -> (w4665:T4)
                    n2510 = local read "SIG LAB05-2"() -> (w4666:T2)
                    n2511 = local read "ON L05-2"() -> (w4662:cluster{"amps":dbl, "volts":dbl, "pf":dbl})
                    n2512 = Unbundle(w4666) -> ("AMPS"=w4672:dbl, "VOLTS"=w4670:dbl, "PF"=w4669:dbl, "Tmp Live"=w4668:dbl, "Tmp Neut"=w4671:dbl)
                    n2513 = Unbundle(w4665) -> ("CYCLE"=w4667:dbl)  [unwired: 2 out]
                    n2514 = stacked-sequence {
                      tunnel: w4672 -> [w4676 w4695]
                      tunnel: w4671 -> [_ w4694]
                      tunnel: w4670 -> [w4675 w4693]
                      tunnel: w4669 -> [w4674 w4692]
                      tunnel: w4668 -> [_ w4691]
                      tunnel: w4667 -> [_ w4690]
                      tunnel: w4664 -> [_ w4689]
                      tunnel: w4663 -> [w4677 _]
                      tunnel: w4662 -> [w4673 w4687]
                      tunnel: w4661 -> [_ w4688]
                      tunnel: w4660 -> [_ w4683]
                      frame #0 {
                        n2515 = case shown="True" w4677 {
                          tunnel: w4676 -> [_ w4682]
                          tunnel: w4675 -> [_ w4681]
                          tunnel: w4674 -> [_ w4680]
                          tunnel: w4673 -> [_ w4678]
                          frame False {
                          }
                          frame True {
